vi "Drop 'Em.vi"(11 "Bricks in":T1(array[cluster])) -> (3 "Bricks out":T1(array[cluster]))   [LabVIEW 2023, in "d22.lvlib"]
uses:
  d22.lvlib
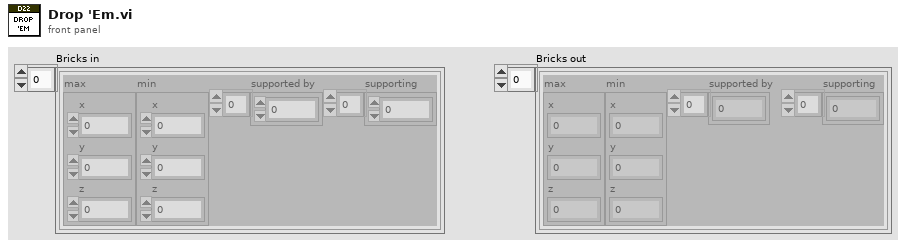
[diagram p1: front panel]
types:
  T1 = cluster{"max":cluster{"x":i32, "y":i32, "z":i32}, "min":cluster{"x":i32, "y":i32, "z":i32}, "supported by":i32[], "supporting":i32[]}[]
  T2 = cluster{"max":cluster{"x":i32, "y":i32, "z":i32}, "min":cluster{"x":i32, "y":i32, "z":i32}, "supported by":i32[], "supporting":i32[]}
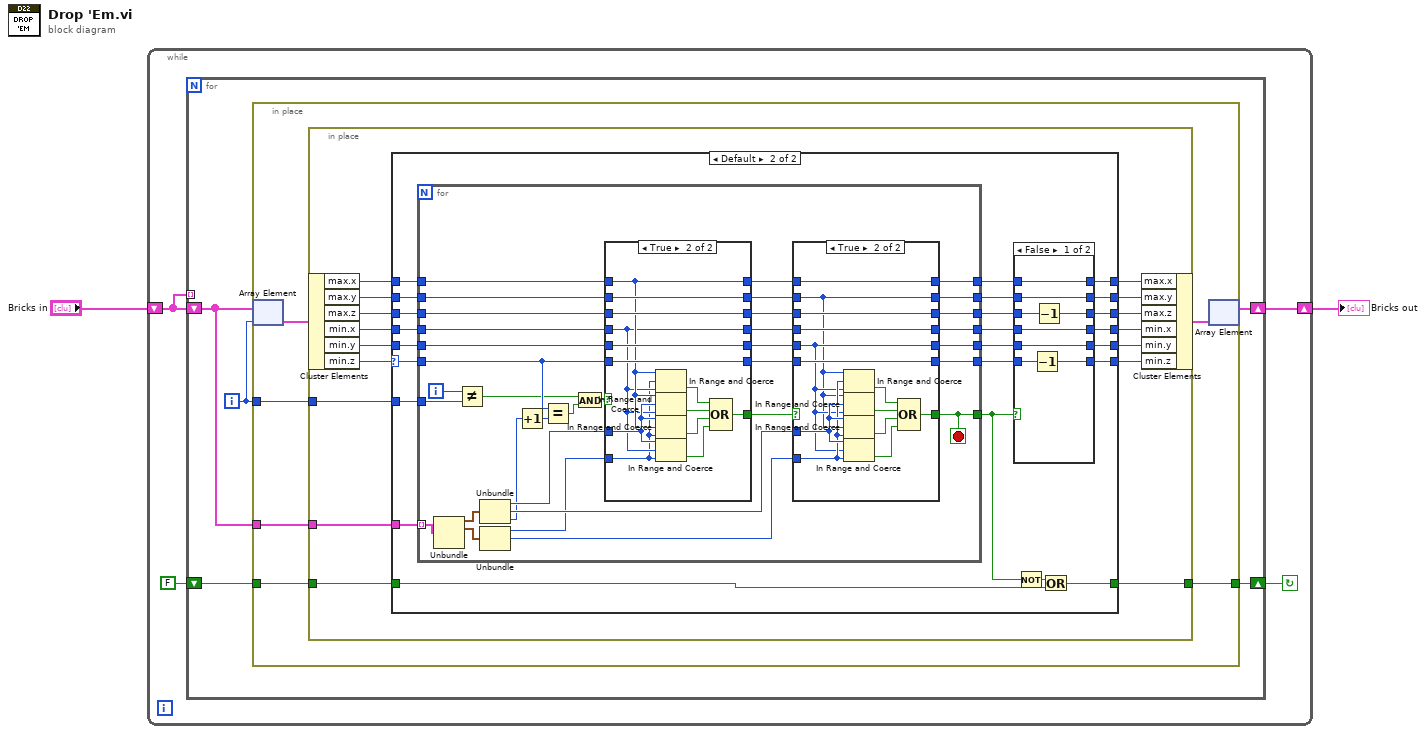
[diagram p0: block diagram]
diagram:
  n1 = while {
    shift-right: [w6] -> w2
    shift-left: "Bricks in" -> [w3]
    stop <- w4 continue-if-true
    n2 = for {
      shift-right: [w7] -> w6
      shift-left: w3 -> [w8]
      shift-right: [w10] -> w4
      shift-left: FALSE -> [w11]
      tunnel: w3 -> [_] mode=indexing
      i -> [w9]
      n3 = in-place {
        in-place-border: w8 -> [w17]
        in-place-border: w11 -> [w14]
        in-place-border: [w13] -> w10
        in-place-border: w9 -> [w12]
        n4 = in-place-array #1(w8, w9) -> (w16:T2)
        n5 = in-place {
          in-place-border: w17 -> [w18]
          in-place-border: w14 -> [w21]
          in-place-border: [w20] -> w13
          in-place-border: w12 -> [w19]
          n6 = in-place-cluster #2(w16) -> ("max.x"=w32:i32, "max.y"=w33:i32, "max.z"=w31:i32, "min.x"=w30:i32, "min.y"=w29:i32, "min.z"=w28:i32)
          n7 = case shown="Default" w28 {
            selector: w28 -> [w35 w58]
            tunnel: w18 -> [_ w64]
            tunnel: w33 -> [w39 w63]
            tunnel: w32 -> [w40 w62]
            tunnel: w30 -> [w37 w60]
            tunnel: w29 -> [w36 w59]
            tunnel: [w40 w51] -> w27
            tunnel: [w39 w50] -> w26
            tunnel: [w38 w49] -> w25
            tunnel: [w37 w48] -> w24
            tunnel: [w36 w47] -> w23
            tunnel: [w35 w46] -> w22
            tunnel: w31 -> [w38 w61]
            tunnel: w21 -> [w34 w45]
            tunnel: [w34 w42] -> w20
            tunnel: w19 -> [_ w41]
            frame 1 {
            }
            frame Default {
              n8 = for {
                tunnel: w64 -> [w112] mode=indexing
                tunnel: w63 -> [w108]
                tunnel: w62 -> [w109]
                tunnel: w61 -> [w107]
                tunnel: w60 -> [w106]
                tunnel: w59 -> [w105]
                tunnel: w58 -> [w103]
                tunnel: [w90] -> w44
                tunnel: [w96] -> w57
                tunnel: [w95] -> w56
                tunnel: [w94] -> w55
                tunnel: [w93] -> w54
                tunnel: [w92] -> w53
                tunnel: [w91] -> w52
                tunnel: w41 -> [w87]
                i -> [w88]
                stop <- w90 stop-if-true
                n9 = Unbundle(w112) -> ("max"=w111:cluster{"x":i32, "y":i32, "z":i32}, "min"=w110:cluster{"x":i32, "y":i32, "z":i32})  [unwired: 2 out]
                n10 = Not Equal?(x=w88, y=w87) -> (x != y?=w85:bool)
                n11 = Unbundle(w111) -> ("x"=w84:i32, "y"=w83:i32, "z"=w81:i32)
                n12 = Unbundle(w110) -> ("x"=w80:i32, "y"=w82:i32)  [unwired: 1 out]
                n13 = Increment(x=w81) -> (x+1=w79:i32)
                n14 = Equal?(x=w103, y=w79) -> (x = y?=w104:bool)
                n15 = And(x=w85, y=w104) -> (x .and. y?=w86:bool)
                n16 = case shown="True" w86 {
                  tunnel: w109 -> [w137 w145]
                  tunnel: w108 -> [w136 w150]
                  tunnel: w107 -> [w135 w149]
                  tunnel: w106 -> [w134 w144]
                  tunnel: w105 -> [w133 w148]
                  tunnel: w103 -> [w132 w147]
                  tunnel: [_ w138] -> w89
                  tunnel: [w137 w145] -> w97
                  tunnel: [w136 w150] -> w98
                  tunnel: [w135 w149] -> w99
                  tunnel: [w134 w144] -> w100
                  tunnel: [w133 w148] -> w101
                  tunnel: [w132 w147] -> w102
                  tunnel: w84 -> [_ w146]
                  tunnel: w80 -> [_ w143]
                  frame False {
                  }
                  frame True {
                    n17 = In Range and Coerce(upper limit=w145, x=w143, lower limit=w144) -> (In Range?=w139:bool)  [unwired: 1 out]
                    n18 = In Range and Coerce(upper limit=w145, x=w146, lower limit=w144) -> (In Range?=w141:bool)  [unwired: 1 out]
                    n19 = In Range and Coerce(upper limit=w146, x=w145, lower limit=w143) -> (In Range?=w142:bool)  [unwired: 1 out]
                    n20 = In Range and Coerce(upper limit=w146, x=w144, lower limit=w143) -> (In Range?=w140:bool)  [unwired: 1 out]
                    n21 = Compound Arithmetic op=OR(w139, w141, w142, w140) -> (w138:bool)
                  }
                }
                n22 = case shown="True" w89 {
                  tunnel: w97 -> [w118 w128]
                  tunnel: w98 -> [w117 w119]
                  tunnel: w99 -> [w116 w131]
                  tunnel: w100 -> [w115 w127]
                  tunnel: w101 -> [w114 w120]
                  tunnel: w102 -> [w113 w130]
                  tunnel: [_ w121] -> w90
                  tunnel: [w118 w128] -> w96
                  tunnel: [w117 w119] -> w95
                  tunnel: [w116 w131] -> w94
                  tunnel: [w115 w127] -> w93
                  tunnel: [w114 w120] -> w92
                  tunnel: [w113 w130] -> w91
                  tunnel: w83 -> [_ w129]
                  tunnel: w82 -> [_ w126]
                  frame False {
                  }
                  frame True {
                    n23 = In Range and Coerce(upper limit=w119, x=w126, lower limit=w120) -> (In Range?=w122:bool)  [unwired: 1 out]
                    n24 = In Range and Coerce(upper limit=w119, x=w129, lower limit=w120) -> (In Range?=w124:bool)  [unwired: 1 out]
                    n25 = In Range and Coerce(upper limit=w129, x=w119, lower limit=w126) -> (In Range?=w125:bool)  [unwired: 1 out]
                    n26 = In Range and Coerce(upper limit=w129, x=w120, lower limit=w126) -> (In Range?=w123:bool)  [unwired: 1 out]
                    n27 = Compound Arithmetic op=OR(w122, w124, w125, w123) -> (w121:bool)
                  }
                }
              }
              n28 = case shown="False" w44 {
                tunnel: w57 -> [w67 w78]
                tunnel: w56 -> [w72 w77]
                tunnel: w55 -> [w71 w76]
                tunnel: w54 -> [w70 w75]
                tunnel: w53 -> [w69 w74]
                tunnel: w52 -> [w68 w73]
                tunnel: [w67 w78] -> w51
                tunnel: [w72 w77] -> w50
                tunnel: [w66 w76] -> w49
                tunnel: [w70 w75] -> w48
                tunnel: [w69 w74] -> w47
                tunnel: [w65 w73] -> w46
                frame False {
                  n29 = Decrement(x=w68) -> (x-1=w65:i32)
                  n30 = Decrement(x=w71) -> (x-1=w66:i32)
                }
                frame True {
                }
              }
              n31 = Not(x=w44) -> (.not. x?=w43:bool)
              n32 = Or(x=w43, y=w45) -> (x .or. y?=w42:bool)
            }
          }
          n33 = in-place-cluster #2("max.x"=w27, "max.y"=w26, "max.z"=w25, "min.x"=w24, "min.y"=w23, "min.z"=w22) -> (w15:T2)
        }
        n34 = in-place-array #1(w15) -> (w7:T1)  [unwired: 1 out]
      }
    }
  }
  "Bricks out" <- w2
